vi "Binomial Noise (obs 90).vi"(2 "seed":i32=-1, 3 "trial probability":dbl=0.5 format="%.2f", 4 "trials":i32=1, 5 "samples":i32=128) -> (0 "error":i32, 1 "binomial noise":u32[](array[numeric]))   [LabVIEW 2020, in "NI_AALBase.lvlib"]
doc: "The Binomial Noise VI was rewritten in LabVIEW 2009. Replace this VI with a Binomial Noise VI from the <B>Functions</B> palette to use the new functionality.\n\nGenerates a binomially-distributed, pseudorandom pattern whose values are the number of occurrences of an event, given the probability of that event occurring and the number of trials."
uses:
  <vilib>/Analysis/NI_AALBase.lvlib
  <resource>/lvanlys.dll
panel:
  # "Binomial Noise"
  # "This VI is obsolete !!!\nYou should replace this VI in your diagram with the Binomial Noise VI."
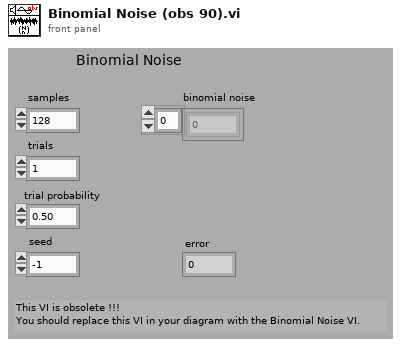
[diagram p1: front panel]
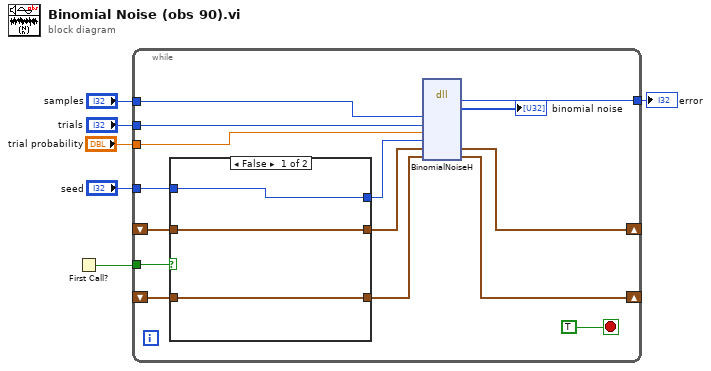
[diagram p0: block diagram]
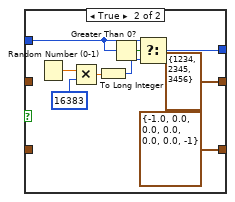
[diagram p2: hidden frame]
diagram:
  n1 = First Call?() -> (First Call?: T/F=w2:bool)
  n2 = while {
    tunnel: [w17] -> w6
    tunnel: "seed" -> [w14]
    tunnel: "trials" -> [w21]
    tunnel: "samples" -> [w20]
    shift-right: [w9] -> _
    shift-left: _ -> [w15]
    shift-right: [w11] -> _
    shift-left: _ -> [w13]
    tunnel: w2 -> [w16]
    tunnel: "trial probability" -> [w7]
    stop <- TRUE stop-if-true
    n3 = case shown="False" w16 {
      tunnel: w15 -> [w24 _]
      tunnel: [w24 cluster{"xSeed":i32, "ySeed":i32, "zSeed":i32} {"xSeed"=1234, "ySeed"=2345, "zSeed"=3456} ("RNGState")] -> w10
      tunnel: [w23 w31] -> w8
      tunnel: w14 -> [w23 w32]
      tunnel: [w22 cluster{dbl, dbl, dbl, dbl, dbl, dbl, i32} {-1.0, 0.0, 0.0, 0.0, 0.0, 0.0, -1}] -> w12
      tunnel: w13 -> [w22 _]
      frame False {
      }
      frame True {
        n4 = Random Number (0-1)() -> (number: 0 to 1=w29:dbl)
        n5 = Multiply(x=w29, y=16383 ("x")) -> (x*y=w30:dbl)
        n6 = To Long Integer(number=w30) -> (32bit integer=w28:i32)
        n7 = Greater Than 0?(x=w32) -> (x > 0?=w33:bool)
        n8 = Select(t=w32, s=w33, f=w28) -> (s? t:f=w31:i32)
      }
    }
    n9 = dll-call lib="e:/builds/penguin/labview/branches/2020/dev/dist/resource/lvanlys.*" fn="BinomialNoiseH"("size"=w20, "numTrials"=w21, "trialProb"=w7, "theSeed"=w8, "rngState"=w10, "binomialState"=w12) -> ("return type"=w17:i32, "binomial noise"=→"binomial noise":u32[], "rngState"=w9:cluster{"xSeed":i32, "ySeed":i32, "zSeed":i32}, "binomialState"=w11:cluster{dbl, dbl, dbl, dbl, dbl, dbl, i32})  [unwired: 7 in, 3 out]
  }
  "error" <- w6
